vi "Event Handler.vi"(0 "uService Template in":refnum<class "Template Internal uService.lvclass">, 5 "Event type":T1=enum."Message", 7 "Item Name":string, 9 "Data":variant, 11 "error in (no error)":errorcluster) -> (4 "uService Template out":refnum<class "Template Internal uService.lvclass">, 15 "error out":errorcluster)   [LabVIEW 2026, in "TALOS.lvlib" / "Template Internal uService.lvlib" / "Template Internal uService.lvclass"]
uses:
  Template Internal uService.lvclass
  Father of all uServices/Father of all uServices/Event Handler Items.ctl
  Ancestor/Ancestor/Ancestor.lvclass/Ancestor.ctl
  FGV/Error Memory/Get Error Description.vi
  Support VIs/Get PC name.vi
  Ancestor/Ancestor/Read ID.vi
  Support VIs/Get Class Name.vi
  <vilib>/Utility/error.llb/Clear Errors.vi
  FGV/Error Memory/Error Memory Core.vi
  <vilib>/AdvancedString/Delimited String to 1D String Array.vi
  <vilib>/AdvancedString/Delimited String to 1D String Array (string).vi
  Support VIs/Circus Root Path.vi
  FGV/Error Memory/Error Crt Lvl checker.vi
  FGV/Error Memory/Error Memory Core.vi/40c8088d-b597-4017-91af-faa98e00292e.vi
  FGV/Error Memory/Error Memory Core.vi/d4a3ab98-063c-4e44-b43d-fbdcfe6c2be2.vi
  Support VIs/Global Memory.vi
  <vilib>/Utility/LVClass/Get LV Class Name.vi
  Support VIs/Is in Packed Library.vi
  Support VIs/TALOS Root path.vi
  Support VIs/Read CSV worksheet.vi
  Support VIs/Global Constants.vi
  <vilib>/Utility/error.llb/General Error Handler.vi
  Ancestor/Ancestor/Ancestor.lvclass
  <vilib>/Comparison/Equal/Equal Functor/Equal Functor.lvclass
  Father of all uServices/Father of all uServices/Father of all uServices.lvclass
  TALOS.lvlib
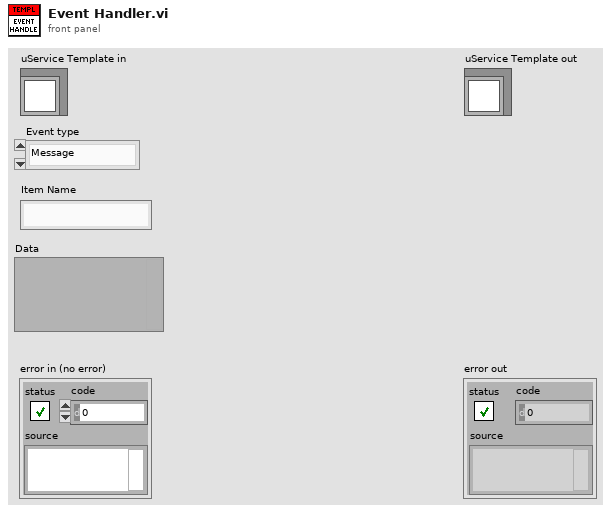
[diagram p1: front panel]
types:
  T1 = typedef "TALOS.lvlib/Father of all uServices.lvlib/Father of all uServices.lvclass/Event Handler Items.ctl" = enum16{"Button Pressed", "Message", "Ready to launch?", "Safe Mode", "Start RUN", "Stop RUN"}
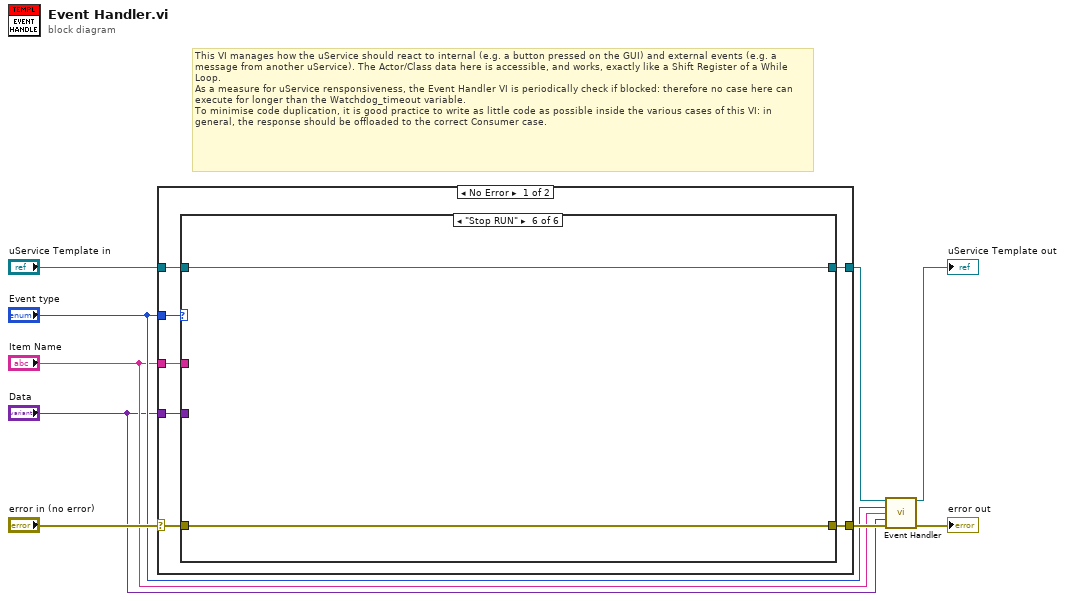
[diagram p0: block diagram]
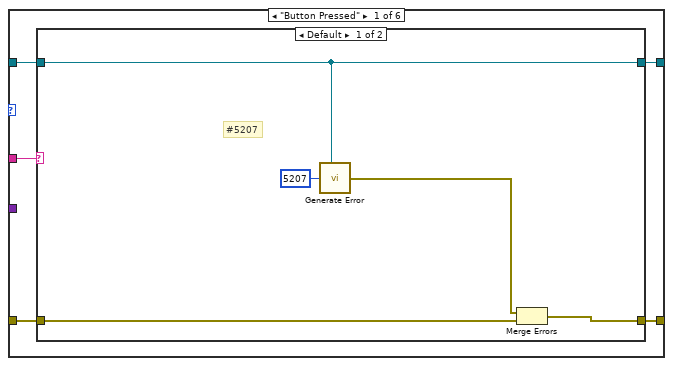
[diagram p2: hidden frame]
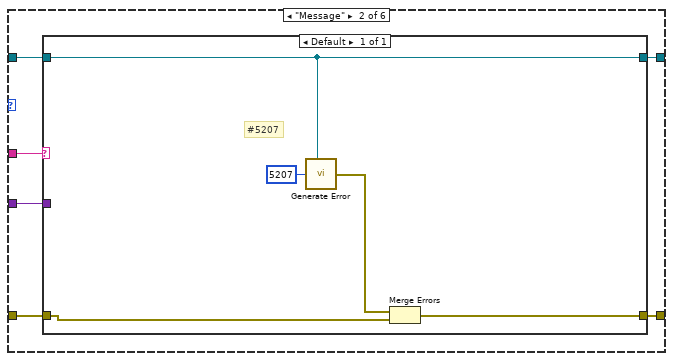
[diagram p4: hidden frame]
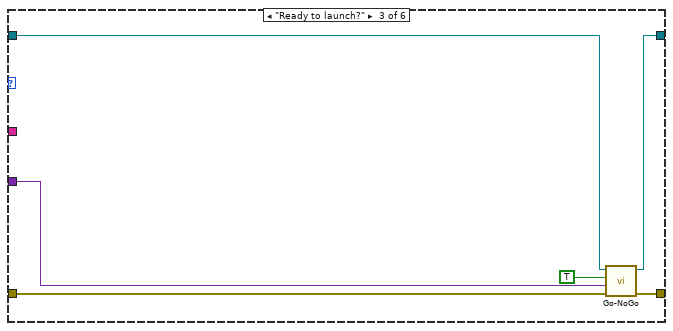
[diagram p5: hidden frame]
diagram:
  # "This VI manages how the uService should react to internal (e.g. a button pressed on the GUI) and external events (e.g. a message from another uService). The Actor/Class data here is accessible, and works, exactly like a Shift Register of a While Loop. \nAs a measure for uService rensponsiveness, the Event Handler VI is periodically check if blocked: therefore no case here can execute for longer than the Watchdog_timeout variable. \nTo minimise code duplication, it is good practice to write as little code as possible inside the various cases of this VI: in general, the response should be offloaded to the correct Consumer case."
  n1 = case shown="No Error" "error in (no error)" {
    selector: "error in (no error)" -> [w13 w53]
    tunnel: [w12 w53] -> w7
    tunnel: "uService Template in" -> [w15 w52]
    tunnel: [w14 w52] -> w4
    tunnel: "Event type" -> [w16 _]
    tunnel: "Item Name" -> [w11 _]
    tunnel: "Data" -> [w10 _]
    frame No Error {
      n2 = case shown="\"Stop RUN\"" w16 {
        tunnel: w15 -> [w21 w34 w42 w47 w49 w51]
        tunnel: [w20 w30 w45 w47 w49 w51] -> w14
        tunnel: w13 -> [w17 w31 w43 w46 w48 w50]
        tunnel: [w18 w29 w44 w46 w48 w50] -> w12
        tunnel: w11 -> [w19 w33 _ _ _ _]
        tunnel: w10 -> [_ w32 w40 _ _ _]
        frame "Button Pressed" {
          n3 = case shown="Default" w19 {
            tunnel: w21 -> [w22 w28]
            tunnel: [w22 w28] -> w20
            tunnel: [w25 w27] -> w18
            tunnel: w17 -> [w26 w27]
            frame Default {
              # "#5207"
              n4 = call "Generate Error.vi"("Class"=w22, "Error Code"=5207) -> ("error out"=w24:errorcluster)  [unwired: 5 in]
              n5 = Merge Errors(w24, w26) -> (w25:errorcluster)
            }
            frame "Example" {
            }
          }
        }
        frame "Message" {
          n6 = case shown="Default" w33 {
            tunnel: w34 -> [w37]
            tunnel: w32 -> [_]
            tunnel: w31 -> [w35]
            tunnel: [w37] -> w30
            tunnel: [w36] -> w29
            frame Default {
              # "#5207"
              n7 = call "Generate Error.vi"("Class"=w37, "Error Code"=5207) -> ("error out"=w38:errorcluster)  [unwired: 5 in]
              n8 = Merge Errors(w38, w35) -> (w36:errorcluster)
            }
          }
        }
        frame "Ready to launch?" {
          n9 = call-dynamic "Go-NoGo.vi"("error in (no error)"=w43, "Go-NoGo Data"=w40, "Go?"=TRUE, "Father of all uServices in"=w42) -> ("error out"=w44:errorcluster, "Father of all uServices out"=w45:refnum<class "Template Internal uService.lvclass">)  [unwired: 6 in]
        }
        frame "Safe Mode" {
        }
        frame "Start RUN" {
        }
        frame "Stop RUN" {
        }
      }
    }
    frame Error {
    }
  }
  n10 = call-parent "Event Handler.vi"("uService Template in"=w4, "Event type"="Event type", "Item Name"="Item Name", "Data"="Data", "error in (no error)"=w7) -> ("uService Template out"=→"uService Template out":refnum<class "Template Internal uService.lvclass">, "error out"=→"error out":errorcluster)  [unwired: 9 in]
